vi "Data to List.vi"(0 "Data String In":string, 11 "error in":errorcluster) -> (4 "GEA List":refnum<k24>, 15 "error out":errorcluster)   [LabVIEW 2014, in "GEA2_Toolkit.lvlib"]
uses:
  library/GEA2_Toolkit.lvlib
  C:/Automation/DLLs/PC Tools .NET/GeaCommunication.dll
  Automation/DLLs/PC Tools .NET/GeaCommunication.dll
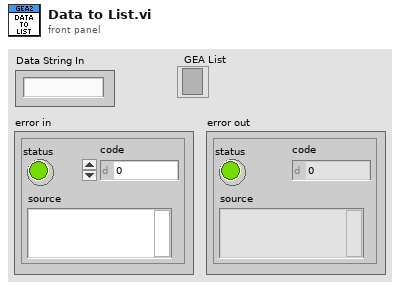
[diagram p1: front panel]
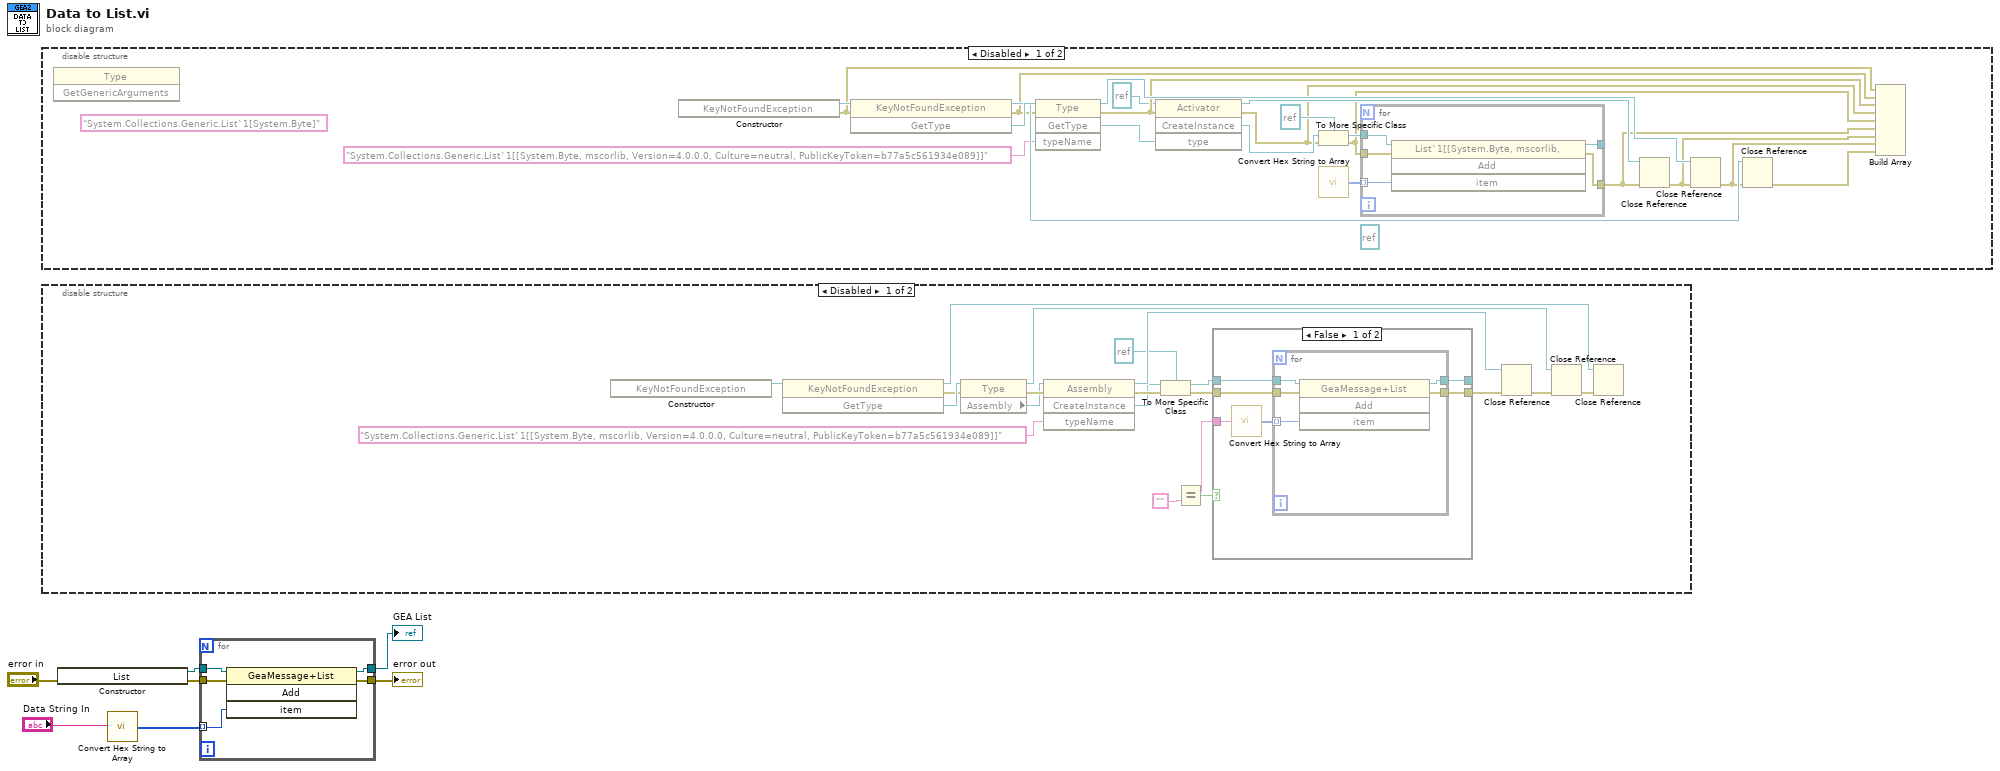
[diagram p0: block diagram]
diagram:
  n1 = disable-structure shown="Disabled" {
    frame Disabled {
      (unwired) "System.Collections.Generic.List`1[System.Byte]" ("typeName")
      (unwired) refnum<k24> refnum ("reference")
      n2 = invoke class="Type" method="GetGenericArguments"() -> ()  [unwired: 3 in, 3 out]
      n3 = constructor class="KeyNotFoundException"() -> (reference out=w21:refnum<k24>, error out=w17:errorcluster)  [unwired: 3 in, 1 out]
      n4 = invoke class="KeyNotFoundException" method="GetType"(reference=w21, error in=w17) -> (reference out=w27:refnum<k24>, error out=w15:errorcluster, "GetType"=w28:refnum<k24>)  [unwired: 1 in]
      n5 = invoke class="Type" method="GetType"(reference=w28, error in=w15, "typeName"="System.Collections.Generic.List`1[[System.Byte, mscorlib, Version=4.0.0.0, Culture=neutral, PublicKeyToken=b77a5c561934e089]]") -> (reference out=w20:refnum<k24>, error out=w13:errorcluster, "GetType"=w26:refnum<k24>)  [unwired: 1 in, 1 out]
      n6 = invoke class="Activator" method="CreateInstance"(reference=refnum<k24> refnum, error in=w13, "type"=w26) -> (reference out=w25:refnum<k24>, error out=w9:errorcluster, "CreateInstance"=w22:refnum<k24>)  [unwired: 1 in, 1 out]
      n7 = To More Specific Class(target class=refnum<k24> refnum ("reference"), reference=w22, error in=w9) -> (specific class reference=w23:refnum<k24>, error out=w10:errorcluster)
      n8 = call "Convert Hex String to Array.vi"() -> ("Hex Array Out"=w8:u8[])  [unwired: 15 in]
      n9 = for {
        tunnel: w8 -> [w32] mode=indexing
        tunnel: w10 -> [w30]
        tunnel: [w31] -> w11
        tunnel: w23 -> [w29]
        tunnel: [w33] -> _
        n10 = invoke class="List`1[[System.Byte, mscorlib, " method="Add"(reference=w29, error in=w30, "item"=w32) -> (reference out=w33:refnum<k24>, error out=w31:errorcluster)  [unwired: 1 in, 2 out]
      }
      n11 = Close Reference(reference=w25, error in (no error)=w11) -> (error out=w14:errorcluster)
      n12 = Close Reference(reference=w20, error in (no error)=w14) -> (error out=w18:errorcluster)
      n13 = Close Reference(reference=w27, error in (no error)=w18) -> (error out=w19:errorcluster)
      n14 = Build Array(w17, w15, w13, w9, w10, w11, w14, w18, w19) -> ()  [unwired: 1 out]
    }
    frame Enabled {
    }
  }
  n15 = disable-structure shown="Disabled" {
    frame Disabled {
      n16 = constructor class="KeyNotFoundException"() -> (reference out=w50:refnum<k24>)  [unwired: 3 in, 2 out]
      n17 = invoke class="KeyNotFoundException" method="GetType"(reference=w50) -> (reference out=w49:refnum<k24>, error out=w47:errorcluster, "GetType"=w48:refnum<k24>)  [unwired: 2 in]
      n18 = property class="Type"(reference=w48, error in=w47) -> (reference out=w46:refnum<k24>, error out=w41:errorcluster, "Assembly"=w39:refnum<k24>)
      n19 = invoke class="Assembly" method="CreateInstance"(reference=w39, error in=w41, "typeName"="System.Collections.Generic.List`1[[System.Byte, mscorlib, Version=4.0.0.0, Culture=neutral, PublicKeyToken=b77a5c561934e089]]") -> (reference out=w42:refnum<k24>, error out=w43:errorcluster, "CreateInstance"=w37:refnum<k24>)  [unwired: 1 in, 1 out]
      n20 = To More Specific Class(target class=refnum<k24> refnum ("reference"), reference=w37, error in=w43) -> (specific class reference=w40:refnum<k24>, error out=w52:errorcluster)
      n21 = Equal?(x=w53, y="") -> (x = y?=w35:bool)
      n22 = case shown="False" w35 {
        tunnel: [w59 w66] -> _
        tunnel: w52 -> [w57 w65]
        tunnel: [w56 w65] -> w45
        tunnel: w40 -> [w55 w66]
        tunnel: [w54 _] -> w53
        frame False {
          n23 = call "Convert Hex String to Array.vi"("Hex String In"=w54) -> ("Hex Array Out"=w58:u8[])  [unwired: 14 in]
          n24 = for {
            tunnel: w58 -> [w60] mode=indexing
            tunnel: w57 -> [w62]
            tunnel: [w63] -> w56
            tunnel: w55 -> [w61]
            tunnel: [w64] -> w59
            n25 = invoke class="GeaMessage+List" method="Add"(reference=w61, error in=w62, "item"=w60) -> (reference out=w64:refnum<k24>, error out=w63:errorcluster)  [unwired: 1 in, 2 out]
          }
        }
        frame True {
        }
      }
      n26 = Close Reference(reference=w42, error in (no error)=w45) -> (error out=w38:errorcluster)
      n27 = Close Reference(reference=w46, error in (no error)=w38) -> (error out=w51:errorcluster)
      n28 = Close Reference(reference=w49, error in (no error)=w51) -> ()  [unwired: 1 out]
    }
    frame Enabled {
    }
  }
  n29 = constructor class="GeaMessage+List"(error in="error in") -> (reference out=w5:refnum<k24>, error out=w4:errorcluster)  [unwired: 2 in, 1 out]
  n30 = call "Convert Hex String to Array.vi"("Hex String In"="Data String In") -> ("Hex Array Out"=w7:u8[])  [unwired: 14 in]
  n31 = for {
    tunnel: w7 -> [w67] mode=indexing
    tunnel: [w68] -> w3
    tunnel: [w69] -> w6
    tunnel: w5 -> [w71]
    tunnel: w4 -> [w70]
    n32 = invoke class="GeaMessage+List" method="Add"(reference=w71, error in=w70, "item"=w67) -> (reference out=w69:refnum<k24>, error out=w68:errorcluster)  [unwired: 1 in, 2 out]
  }
  "GEA List" <- w6
  "error out" <- w3
